vi "Execute.vi"(8 "error in (no error)":errorcluster, 9 "System in":refnum<class "System.lvclass">, 10 "Command in":refnum<class "Command.lvclass">, 11 "CT-De-Energized-State in":refnum<class "CT-De-Energized-State.lvclass">) -> (0 "error out":errorcluster, 2 "Next State":refnum<class "State.lvclass">, 3 "CT-De-Energized-State out":refnum<class "CT-De-Energized-State.lvclass">)   [LabVIEW 2013, in "CT-De-Energized-State.lvclass"]
uses:
  CT-De-Energized-State.lvclass
  Commands/Command/Command.lvclass
  Systems/System/System.lvclass
  State/State.lvclass
  Systems/Catapult/Catapult.lvclass
  CT-Energizing-State/CT-Energizing-State.lvclass
  Commands/CT-De-energizeThenStop-Command/CT-De-energizeThenStop-Cmd.lvclass
  CT-Stopping-State/CT-Stopping-State.lvclass
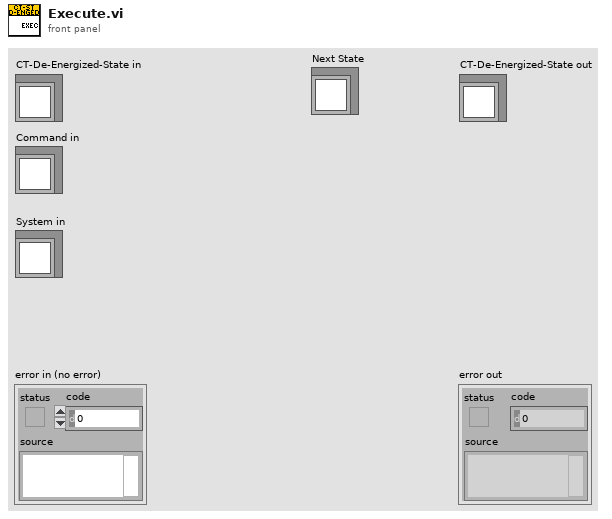
[diagram p1: front panel]
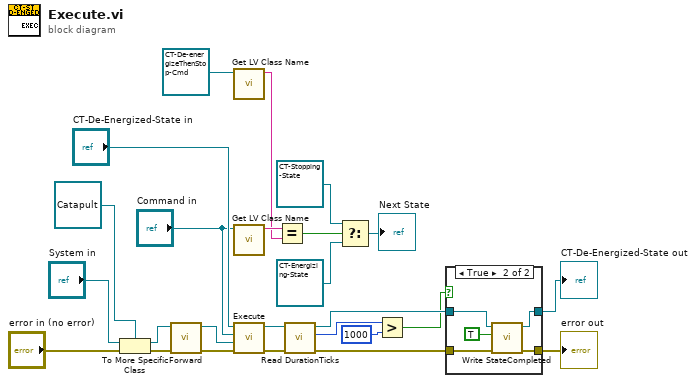
[diagram p0: block diagram]
diagram:
  n1 = To More Specific Class(target class=refnum<class "Catapult.lvclass"> refnum ("Catapult.lvclass"), reference="System in", error in="error in (no error)") -> (specific class reference=w19:refnum<class "Catapult.lvclass">, error out=w9:errorcluster)
  n2 = call-dynamic "Forward.vi"("error in (no error)"=w9, "Catapult in"=w19) -> ("error out"=w10:errorcluster, "Catapult out"=w11:refnum<class "Catapult.lvclass">)  [unwired: 8 in]
  n3 = call <vilib>:"Get LV Class Name.vi"("object"=refnum<class "CT-De-energizeThenStop-Cmd.lvclass"> refnum ("CT-De-energizeThenStop-Cmd.lvclass")) -> ("class name"=w5:string)  [unwired: 9 in, 1 out]
  n4 = call <vilib>:"Get LV Class Name.vi"("object"="Command in") -> ("class name"=w6:string)  [unwired: 9 in, 1 out]
  n5 = call-parent "Execute.vi"("error in (no error)"=w10, "System in"=w11, "Command in"="Command in", "State in"="CT-De-Energized-State in") -> ("error out"=w16:errorcluster, "State out"=w18:refnum<class "CT-De-Energized-State.lvclass">)  [unwired: 5 in, 1 out]
  n6 = Equal?(x=w6, y=w5) -> (x = y?=w4:bool)
  n7 = call "Read DurationTicks.vi"("error in (no error)"=w16, "State in"=w18) -> ("error out"=w15:errorcluster, "DurationTicks"=w14:u32, "State out"=w17:refnum<class "CT-De-Energized-State.lvclass">)  [unwired: 7 in]
  n8 = Select(t=refnum<class "CT-Stopping-State.lvclass"> refnum ("CT-Stopping-State.lvclass"), s=w4, f=refnum<class "CT-Energizing-State.lvclass"> refnum ("CT-Energizing-State.lvclass")) -> (s? t:f=→"Next State":refnum<class "State.lvclass">)
  n9 = Greater?(x=w14, y=u32 1000) -> (0:w12:bool)
  n10 = case shown="True" w12 {
    tunnel: [w27 w32] -> w21
    tunnel: [w26 w30] -> w20
    tunnel: w17 -> [w27 w29]
    tunnel: w15 -> [w26 w28]
    frame False {
    }
    frame True {
      n11 = call-dynamic "Write StateCompleted.vi"("error in (no error)"=w28, "StateCompleted"=TRUE, "State in"=w29) -> ("error out"=w30:errorcluster, "State out"=w32:refnum<class "CT-De-Energized-State.lvclass">)  [unwired: 7 in]
    }
  }
  "error out" <- w20
  "CT-De-Energized-State out" <- w21
